vi "FTW-dotNET-SQL-ConnectionEventsCallback.vi"(4 "SQL DB Message":refnum<user-event>, 5 "Event Data":cluster{"sender":refnum<k24>, "e":refnum<k24>}, 6 "Control Ref":refnum<k24>, 7 "Event Common Data":T1) -> ()   [LabVIEW 2015]
uses:
  System.Data
panel:
  # "Inputs"
  # "Outputs"
  # "Callback VI has no outputs"
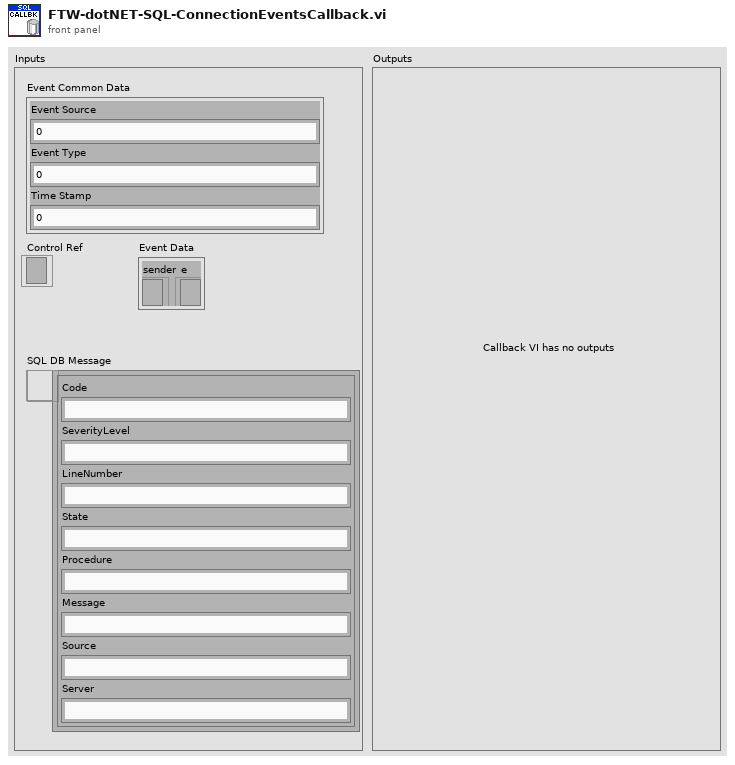
[diagram p1: front panel]
types:
  T1 = cluster{"Event Source":i32, "Event Type":u32, "Time Stamp":u32}
  T2 = cluster{"Code":i32, "SeverityLevel":i32, "LineNumber":i32, "State":i32, "Procedure":string, "Message":string, "Source":string, "Server":string}
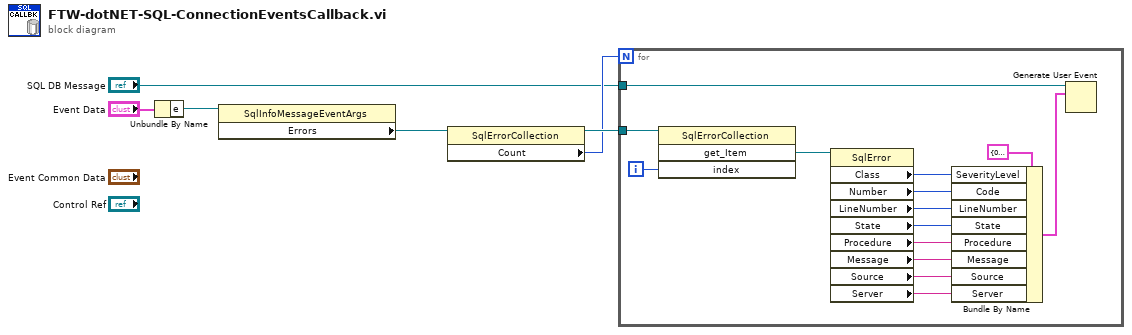
[diagram p0: block diagram]
diagram:
  n1 = Unbundle By Name("Event Data") -> ("e"=w5:refnum<k24>)
  n2 = property class="SqlInfoMessageEventArgs"(reference=w5) -> ("Errors"=w4:refnum<k24>)  [unwired: 1 in, 2 out]
  n3 = property class="SqlErrorCollection"(reference=w4) -> (reference out=w3:refnum<k24>, "Count"=w2:i32)  [unwired: 1 in, 1 out]
  n4 = for {
    N: w2 -> [_]
    tunnel: w3 -> [w16]
    tunnel: "SQL DB Message" -> [w19]
    i -> [w15]
    n5 = invoke class="SqlErrorCollection" method="get_Item"(reference=w16, "index"=w15) -> ("get_Item"=w20:refnum<k24>)  [unwired: 2 in, 3 out]
    n6 = property class="SqlError"(reference=w20) -> ("Class"=w14:u8, "Number"=w13:i32, "LineNumber"=w12:i32, "State"=w11:u8, "Procedure"=w10:string, "Message"=w9:string, "Source"=w7:string, "Server"=w8:string)  [unwired: 1 in, 2 out]
    n7 = Bundle By Name(cluster=T2 {"Code"=0, "SeverityLevel"=0, "LineNumber"=0, "State"=0, "Procedure"="", "Message"="", "Source"="", "Server"=""} ("event data"), "SeverityLevel"=w14, "Code"=w13, "LineNumber"=w12, "State"=w11, "Procedure"=w10, "Message"=w9, "Source"=w7, "Server"=w8) -> (w17:T2)
    n8 = Generate User Event(user event=w19, event data cluster=w17) -> ()  [unwired: 2 in, 2 out]
  }
